vi "Delete Tree Priv.vi"(8 "Error In":errorcluster, 10 "Unique ID":string, 11 "Tree Dictionary In":variant) -> (0 "Error Out":errorcluster, 3 "Tree Dictionary Out":variant)   [LabVIEW 2016, in "Tree Manager.lvclass"]
uses:
  Tree Manager.lvclass
  Typedefs/Tree.ctl
  <vilib>/Utility/error.llb/Error Cluster From Error Code.vi
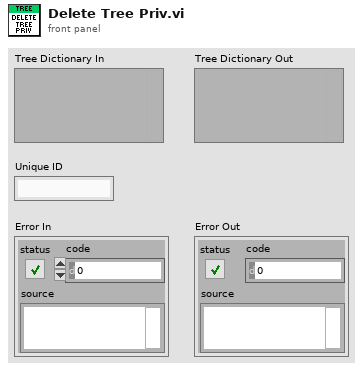
[diagram p1: front panel]
types:
  T1 = typedef "Tree Manager.lvclass/Tree.ctl" = cluster{"Unique ID":string, "Parent ID":string, "Child IDs":string[], "Data":variant, "Name":string}
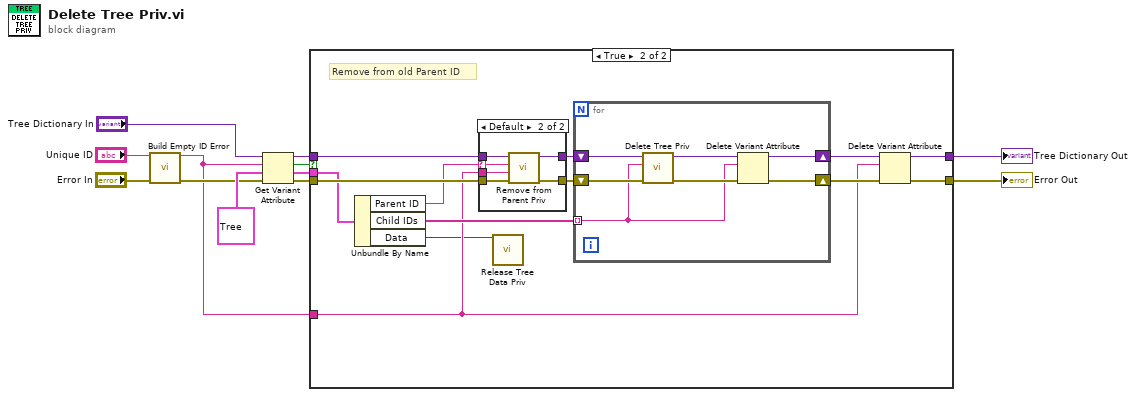
[diagram p0: block diagram]
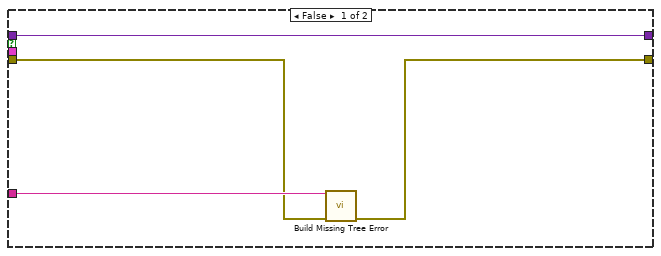
[diagram p2: hidden frame]
diagram:
  n1 = call "Build Empty ID Error.vi"("Unique ID"="Unique ID", "Error In"="Error In") -> ("Unique ID Out"=w1:string, "Error Out"=w2:errorcluster)  [unwired: 12 in]
  n2 = Get Variant Attribute(Variant="Tree Dictionary In", name=w1, default value (empty Variant)=T1 {"Unique ID"="", "Parent ID"="", "Child IDs"=[], "Data"=variant, "Name"=""} ("Cluster of class private data"), error in=w2) -> (duplicate Variant=w7:variant, found=w9:bool, value=w8:T1, error out=w6:errorcluster)
  n3 = case shown="True" w9 {
    tunnel: w8 -> [_ w28]
    tunnel: w7 -> [w16 w27]
    tunnel: w6 -> [w13 w29]
    tunnel: [w14 w21] -> w11
    tunnel: [w16 w20] -> w12
    tunnel: w1 -> [w15 w19]
    frame False {
      n4 = call "Build Missing Tree Error.vi"("Unique ID"=w15, "Error In"=w13) -> ("Error Out"=w14:errorcluster)  [unwired: 13 in]
    }
    frame True {
      # "Remove from old Parent ID"
      n5 = Unbundle By Name(w28) -> ("Parent ID"=w17:string, "Child IDs"=w24:string[], "Data"=w18:variant)
      n6 = case shown="Default" w17 {
        selector: w17 -> [_ w32]
        tunnel: w29 -> [w30 w37]
        tunnel: w27 -> [w31 w36]
        tunnel: [w31 w35] -> w26
        tunnel: [w30 w34] -> w25
        tunnel: w19 -> [_ w33]
        frame "" {
        }
        frame Default {
          n7 = call "Remove from Parent Priv.vi"("Error In"=w37, "Unique ID"=w33, "Parent ID"=w32, "Tree Dictionary"=w36) -> ("Error Out"=w34:errorcluster, "Tree Dictionary Out"=w35:variant)  [unwired: 6 in]
        }
      }
      n8 = call "Release Tree Data Priv.vi"("Data"=w18) -> ()  [unwired: 15 in]
      n9 = for {
        shift-right: [w39] -> w22
        shift-left: w25 -> [w43]
        shift-right: [w38] -> w23
        shift-left: w26 -> [w44]
        tunnel: w24 -> [w40] mode=indexing
        n10 = call "Delete Tree Priv.vi"("Error In"=w43, "Unique ID"=w40, "Tree Dictionary In"=w44) -> ("Error Out"=w41:errorcluster, "Tree Dictionary Out"=w42:variant)  [unwired: 7 in]
        n11 = Delete Variant Attribute(4:w41, 6:w40, 7:w42) -> (0:w39:errorcluster, 3:w38:variant)  [unwired: 1 out]
      }
      n12 = Delete Variant Attribute(4:w22, 6:w19, 7:w23) -> (0:w21:errorcluster, 3:w20:variant)  [unwired: 1 out]
    }
  }
  "Tree Dictionary Out" <- w12
  "Error Out" <- w11
